vi "TestLabActor.vi"() -> ()   [LabVIEW 2019]
uses:
  Controllers/TestLabActor/TestLabActor.lvclass
  C:/Program Files/National Instruments/LabVIEW 2019/vi.lib/ActorFramework/Actor/Actor.lvclass
  <vilib>/ActorFramework/Message Enqueuer/Message Enqueuer.lvclass/Message Enqueuer.ctl
  <vilib>/ActorFramework/Message Enqueuer/Enqueue.vi
  Template Module Messages/Open Front Panel Msg/Open Front Panel Msg.lvclass
  C:/Program Files/National Instruments/LabVIEW 2019/vi.lib/ActorFramework/Message/Message.lvclass
  <vilib>/ActorFramework/Stop Msg/Stop Msg.lvclass
  <vilib>/ActorFramework/Message Priority Queue/Priority Enqueue.vi
  <vilib>/ActorFramework/Actor/Actor.lvclass
panel:
  in  "Milliseconds To Wait":i32=2000
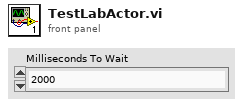
[diagram p1: front panel]
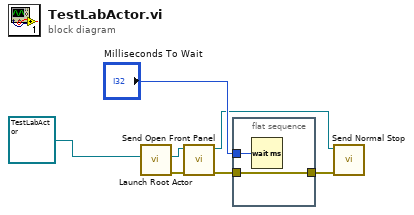
[diagram p0: block diagram]
diagram:
  n1 = call <vilib>:"Launch Root Actor.vi"("Actor"=refnum<class "TestLabActor.lvclass"> refnum ("TestLabActor.lvclass")) -> ("error out"=w7:errorcluster, "Actor's Enqueuer"=w6:refnum<class "Message Enqueuer.lvclass">)  [unwired: 9 in]
  n2 = call "Send Open Front Panel.vi"("error in (no error)"=w7, "Message Enqueuer"=w6) -> ("error out"=w4:errorcluster, "Message Enqueuer out"=w2:refnum<class "Message Enqueuer.lvclass">)  [unwired: 8 in]
  n3 = flat-sequence {
    tunnel: "Milliseconds To Wait" -> [w9]
    tunnel: w4 -> [w8]
    tunnel: [w8] -> w3
    frame #0 {
      n4 = Wait (ms)(milliseconds to wait=w9) -> ()  [unwired: 1 out]
    }
  }
  n5 = call <vilib>:"Send Normal Stop.vi"("error in (no error)"=w3, "Message Enqueuer"=w2) -> ()  [unwired: 9 in, 1 out]
